vi "WriteSCPICommand.vi"(8 "Error In":errorcluster, 10 "SCPI Command":string, 11 "Keithley 6482 In":refnum<visa-resource-name>) -> (0 "Error Out":errorcluster, 3 "Keithley 6482 Out":refnum<visa-resource-name>)   [LabVIEW 2010, in "Keithley-6482-Visa.lvlib"]
uses:
  <instrlib>/lib-labview-8.6-export/Keithley-6482-Visa.lvlib
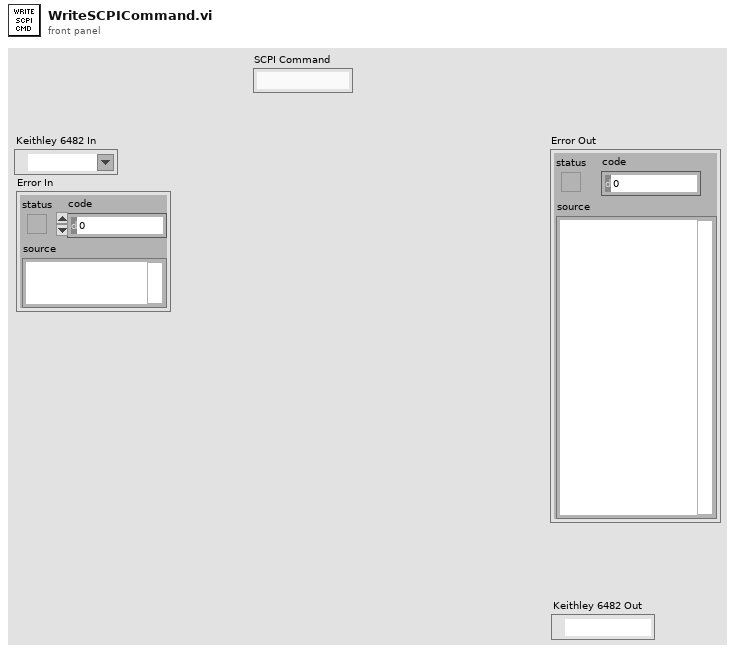
[diagram p1: front panel]
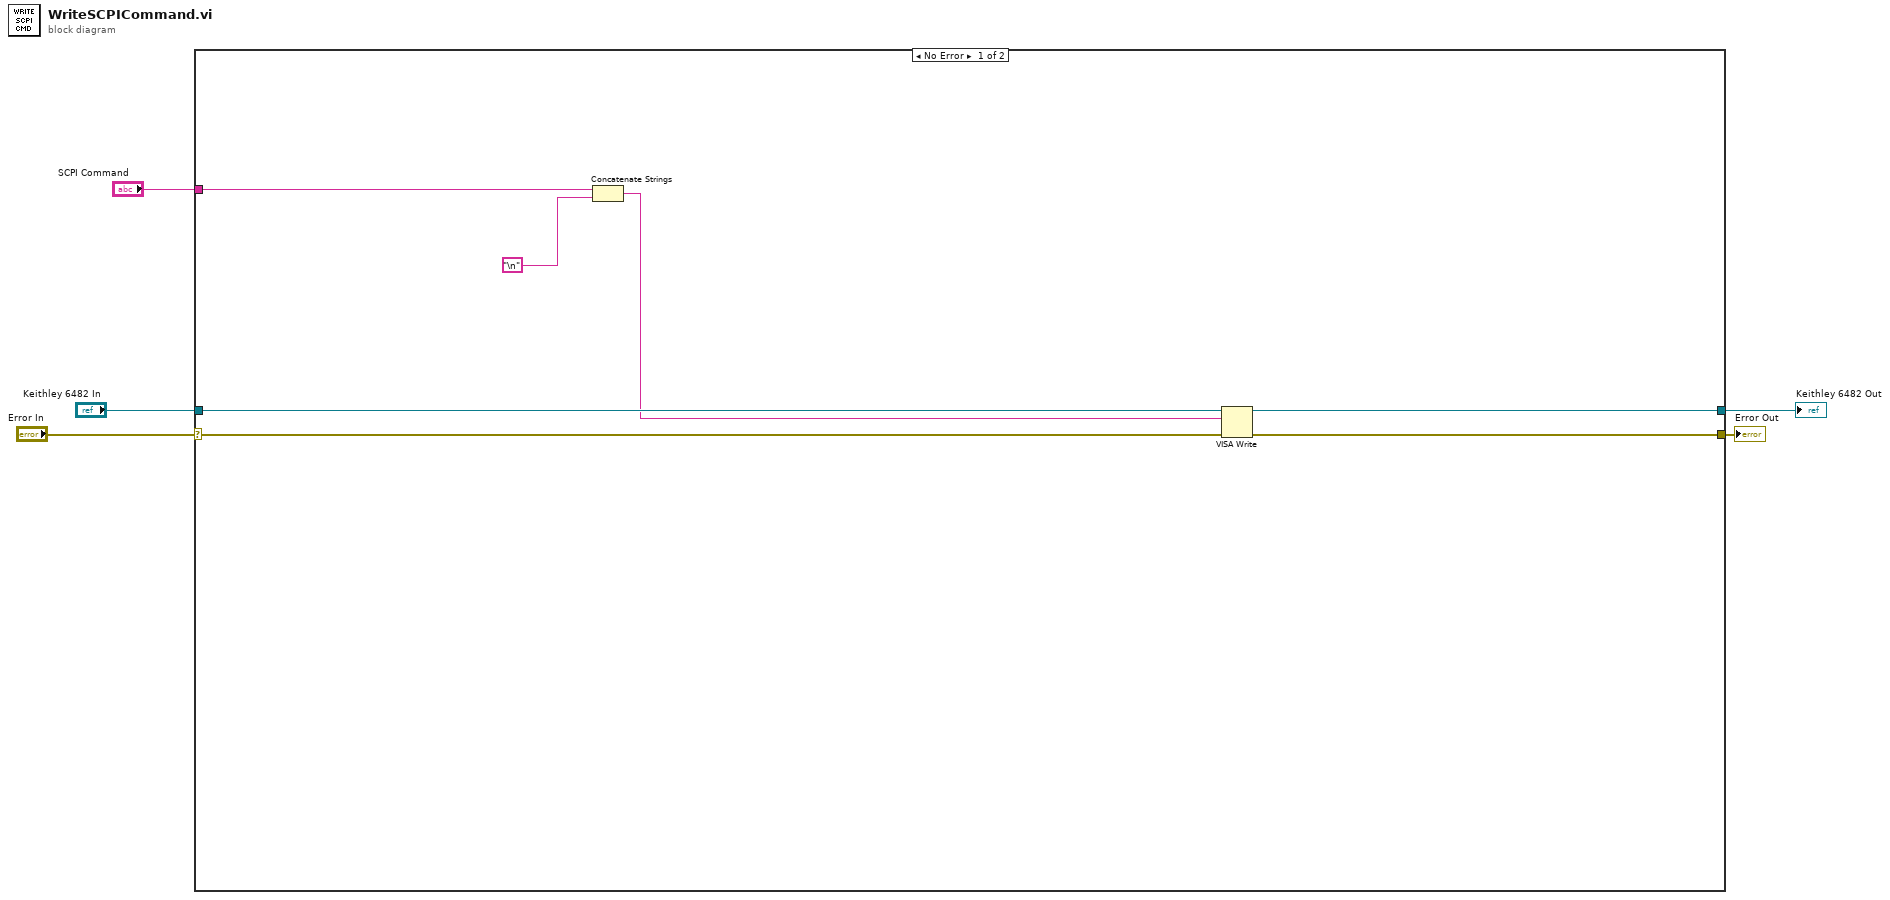
[diagram p0: block diagram]
diagram:
  n1 = case shown="No Error" "Error In" {
    selector: "Error In" -> [w11 w13]
    tunnel: "Keithley 6482 In" -> [w12 w14]
    tunnel: [w10 w13] -> w3
    tunnel: [w9 w14] -> w2
    tunnel: "SCPI Command" -> [w6 _]
    frame No Error {
      n2 = Concatenate Strings(w6, "\n") -> (w8:string)
      n3 = VISA Write(VISA resource name=w12, write buffer=w8, error in (no error)=w11) -> (VISA resource name out=w9:refnum<visa-resource-name>, error out=w10:errorcluster)  [unwired: 1 out]
    }
    frame Error {
    }
  }
  "Error Out" <- w3
  "Keithley 6482 Out" <- w2
